vi "SRV_README.vi"   [LabVIEW 2009]
doc: "Contains all the code for the SRV application. <B>This VI is not intended to be run.</B>\n\n\nAuthor: Mike Schultz - Logic PD"
uses:
  SRV VIs/PacketMode/SRV_PM_Packet.ctl
  SRV VIs/TCP_Communication/SRV_TCP Settings.ctl
  SRV VIs/TCP_Communication/SRV_Package Methods.ctl
  SRV VIs/Support/SRV_Command-Data Queue Data Type.ctl
  SRV VIs/ImageProcessing/QT_Image.ctl
  SRV VIs/SubVIs/SRVGlobals.vi
panel:
  # "SRV\nREADME"
types:
  T1 = typedef "SRV_TCP Settings.ctl" = cluster{"Method":T2, "bytes to read":i32, "timeout ms (1000)":i32}
  T2 = typedef "SRV_Package Methods.ctl" = enum16{"General", "Standard", "CRLF", "Image", "HTML"}
  T3 = typedef "Semaphore RefNum" = refnum<k1>
  T4 = typedef "QT_Image.ctl" = cluster{"Witdh":i32, "Height":i32, "Depth":i32, "data":u8[], "Compressed data":u8[], "Color table":u32[], "Duration":i32, "Options":i32, "Timestamp":i32, "ID":i32, "Reserved":i32, "Dialogs":u32}
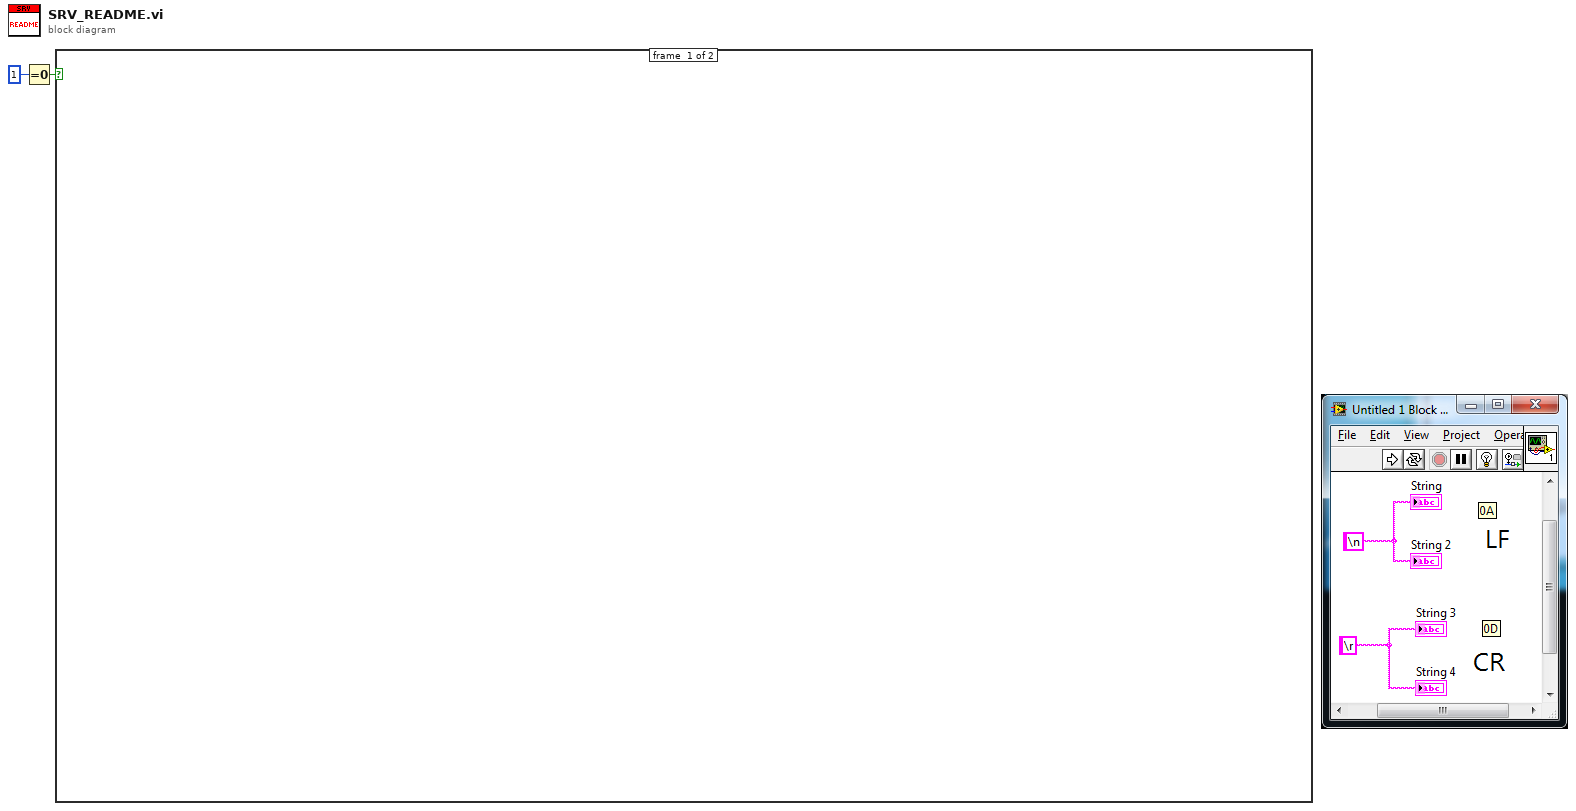
[diagram p0: block diagram]
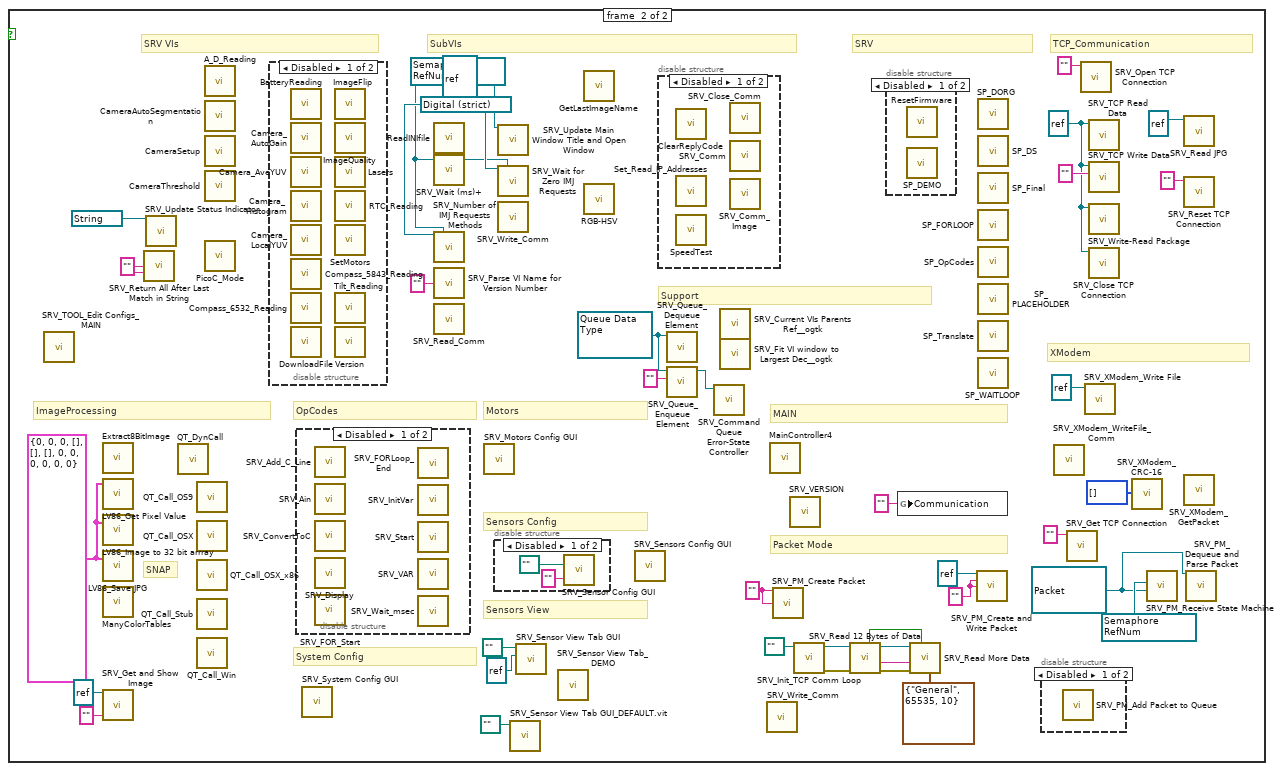
[diagram p2: hidden frame]
diagram:
  n1 = Equal To 0?(x=1) -> (x = 0?=w1:bool)
  n2 = case shown="True" w1 {
    frame #0 {
    }
    frame #1 {
      w6 = refnum<queue> refnum ("SRV_Packets queue")
      w10 = T3 refnum items=["semaphore"] ("TCP Read semaphore")
      w13 = "" ("Command Type")
      w15 = "" ("Command Type")
      w23 = T3 refnum items=["semaphore"] ("semaphore ref")
      w26 = refnum<k5> refnum ("connection ID in")
      w31 = "" ("Reply to XModem Upload")
      w33 = refnum<vi> refnum ("Number of IMJ Requests ref")
      w38 = refnum<queue> refnum ("Command-Data Queue")
      w39 = T4 {"Witdh"=0, "Height"=0, "Depth"=0, "data"=[], "Compressed data"=[], "Color table"=[], "Duration"=0, "Options"=0, "Timestamp"=0, "ID"=0, "Reserved"=0, "Dialogs"=0} ("Image")
      # "SNAP"
      # "MAIN"
      # "System Config"
      # "Sensors View"
      # "Sensors Config"
      # "Motors"
      # "Packet Mode"
      # "TCP_Communication"
      # "XModem"
      # "Support"
      # "SRV"
      # "SubVIs"
      # "SRV VIs"
      # "OpCodes"
      # "ImageProcessing"
      n3 = call "SRV_TOOL_Edit Configs_MAIN.vi"() -> ()  [unwired: 11 in, 1 out]
      n4 = call "Extract8BitImage.vi"() -> ()  [unwired: 2 in, 2 out]
      n5 = call "LV86_Get Pixel Value.vi"("Image In"=w39) -> ()  [unwired: 2 in, 3 out]
      n6 = call "LV86_Image to 32 bit arrray.vi"("Image In"=w39) -> ()  [unwired: 1 in, 2 out]
      n7 = call "LV86_Save JPG.vi"("Image"=w39) -> ()  [unwired: 2 in, 1 out]
      n8 = call "ManyColorTables.vi"() -> ()  [unwired: 3 in, 1 out]
      n9 = call "SRV_Get and Show Image.vi"("Connection ID"=refnum<k5> refnum, "Data"="") -> ()  [unwired: 9 in, 5 out]
      n10 = call "SRV_Return All After Last Match in String.vi"("String"=w31, "String to Match"=w31) -> ()  [unwired: 13 in, 1 out]
      n11 = call "SRV_Update Status Indicator.vi"("Status ref"=refnum<vi> refnum) -> ()  [unwired: 13 in, 2 out]
      n12 = call "QT_DynCall.vi"() -> ()  [unwired: 12 in, 16 out]
      n13 = call "QT_Call_OS9.vi"() -> ()  [unwired: 13 in, 7 out]
      n14 = call "QT_Call_OSX.vi"() -> ()  [unwired: 13 in, 7 out]
      n15 = call "QT_Call_OSX_x86.vi"() -> ()  [unwired: 13 in, 7 out]
      n16 = call "QT_Call_Stub.vi"() -> ()  [unwired: 13 in, 7 out]
      n17 = call "QT_Call_Win.vi"() -> ()  [unwired: 13 in, 7 out]
      n18 = call "A_D_Reading.vi"() -> ()  [unwired: 8 in, 4 out]
      n19 = call "CameraAutoSegmentation.vi"() -> ()  [unwired: 10 in, 2 out]
      n20 = call "CameraSetup.vi"() -> ()  [unwired: 10 in, 2 out]
      n21 = call "CameraThreshold.vi"() -> ()  [unwired: 10 in, 2 out]
      n22 = call "PicoC_Mode.vi"() -> ()  [unwired: 10 in, 2 out]
      n23 = disable-structure shown="Disabled" {
        frame #0 {
          n24 = call "BatteryReading.vi"() -> ()  [unwired: 3 in, 2 out]
          n25 = call "Camera_AutoGain.vi"() -> ()  [unwired: 3 in, 2 out]
          n26 = call "Camera_AveYUV.vi"() -> ()  [unwired: 3 in, 2 out]
          n27 = call "Camera_Histogram.vi"() -> ()  [unwired: 4 in, 1 out]
          n28 = call "Camera_LocalYUV.vi"() -> ()  [unwired: 3 in, 2 out]
          n29 = call "Compass_5843_Reading.vi"() -> ()  [unwired: 3 in, 2 out]
          n30 = call "Compass_6532_Reading.vi"() -> ()  [unwired: 3 in, 2 out]
          n31 = call "DownloadFile.vi"() -> ()  [unwired: 10 in, 2 out]
          n32 = call "ImageFlip.vi"() -> ()  [unwired: 4 in, 1 out]
          n33 = call "ImageQuality.vi"() -> ()  [unwired: 4 in, 1 out]
          n34 = call "Lasers.vi"() -> ()  [unwired: 4 in, 1 out]
          n35 = call "RTC_Reading.vi"() -> ()  [unwired: 3 in, 2 out]
          n36 = call "SetMotors.vi"() -> ()  [unwired: 5 in, 2 out]
          n37 = call "Tilt_Reading.vi"() -> ()  [unwired: 3 in, 2 out]
          n38 = call "Version.vi"() -> ()  [unwired: 8 in, 4 out]
        }
        frame #1 {
        }
      }
      n39 = disable-structure shown="Disabled" {
        frame #0 {
          n40 = call "SRV_Add_C_Line.vi"() -> ()  [unwired: 5 in, 1 out]
          n41 = call "SRV_Ain.vi"() -> ()  [unwired: 3 in, 2 out]
          n42 = call "SRV_ConvertToC.vi"() -> ()  [unwired: 2 in, 2 out]
          n43 = call "SRV_Display.vi"() -> ()  [unwired: 4 in, 1 out]
          n44 = call "SRV_FOR_Start.vi"() -> ()  [unwired: 3 in, 2 out]
          n45 = call "SRV_FORLoop_End.vi"() -> ()  [unwired: 4 in, 1 out]
          n46 = call "SRV_InitVar.vi"() -> ()  [unwired: 2 in, 1 out]
          n47 = call "SRV_Start.vi"() -> ()  [unwired: 4 in, 1 out]
          n48 = call "SRV_VAR.vi"() -> ()  [unwired: 3 in, 4 out]
          n49 = call "SRV_Wait_msec.vi"() -> ()  [unwired: 4 in, 1 out]
        }
        frame #1 {
        }
      }
      n50 = call "SRV_System Config GUI.vi"() -> ()  [unwired: 9 in, 3 out]
      n51 = call "ReadINIfile.vi"() -> ()  [unwired: 9 in, 3 out]
      n52 = call "SRV_Wait (ms)+.vi"() -> ()  [unwired: 14 in, 2 out]
      n53 = call "SRV_Number of IMJ Requests Methods.vi"("Number of IMJ Requests ref"=w33, "semaphore ref"=w23) -> ()  [unwired: 9 in, 5 out]
      n54 = call "SRV_Parse VI Name for Version Number.vi"("VI Name"="") -> ()  [unwired: 14 in, 1 out]
      n55 = call "SRV_Read_Comm.vi"() -> ()  [unwired: 9 in, 3 out]
      n56 = call "SRV_Motors Config GUI.vi"() -> ()  [unwired: 9 in, 3 out]
      n57 = disable-structure shown="Disabled" {
        frame #0 {
          n58 = call "SRV_Sensor Config GUI.vi"("Sensor to Edit"="", "Sensors Config File Path in"=path "") -> ()  [unwired: 7 in, 3 out]
        }
        frame #1 {
        }
      }
      n59 = call "SRV_Update Main Window Title and Open Window.vi"("VI ref"=refnum<vi> refnum) -> ()  [unwired: 13 in, 2 out]
      n60 = call "SRV_Wait for Zero IMJ Requests.vi"("Number of IMJ Requests ref"=w33, "#IMJ semaphore ref"=w23) -> ()  [unwired: 11 in, 3 out]
      n61 = call "SRV_Write_Comm.vi"() -> ()  [unwired: 9 in, 3 out]
      n62 = call "SRV_Sensor View Tab GUI_DEFAULT.vit"("Sensors Config File Path"=path "") -> ()  [unwired: 10 in, 1 out]
      n63 = call "SRV_Sensor View Tab GUI.vi"("SRV In"=refnum<k5> refnum, "Sensors Config File Path"=path "") -> ()  [unwired: 9 in, 1 out]
      n64 = call "SRV_Sensor View Tab_DEMO.vi"() -> ()  [unwired: 1 in]
      n65 = call "GetLastImageName.vi"() -> ()  [unwired: 1 in, 1 out]
      n66 = call "RGB-HSV.vi"() -> ()  [unwired: 14 in, 2 out]
      n67 = call "SRV_Sensors Config GUI.vi"() -> ()  [unwired: 9 in, 3 out]
      n68 = disable-structure shown="Disabled" {
        frame #0 {
          n69 = call "ClearReplyCode.vi"() -> ()  [unwired: 1 in, 1 out]
          n70 = call "Set_Read_IP_Addresses.vi"() -> ()  [unwired: 3 in, 1 out]
          n71 = call "SpeedTest.vi"() -> ()  [unwired: 1 in]
          n72 = call "SRV_Close_Comm.vi"() -> ()  [unwired: 9 in, 3 out]
          n73 = call "SRV_Comm.vi"() -> ()  [unwired: 3 in, 3 out]
          n74 = call "SRV_Comm_Image.vi"() -> ()  [unwired: 3 in, 3 out]
        }
        frame #1 {
        }
      }
      n75 = call "SRV_Queue_Dequeue Element.vi"("Command-Data Queue"=w38) -> ()  [unwired: 5 in, 6 out]
      n76 = call "SRV_Queue_Enqueue Element.vi"("Command"="", "Command-Data Queue"=w38) -> ("Command-Data Queue out"=w22:refnum<queue>)  [unwired: 7 in, 2 out]
      n77 = call "SRV_Command Queue Error-State Controller.vi"("Command-Data Queue"=w22) -> ()  [unwired: 9 in, 2 out]
      n78 = call "SRV_Current VIs Parents Ref__ogtk.vi"() -> ()  [unwired: 2 in, 1 out]
      n79 = call "SRV_Fit VI window to Largest Dec__ogtk.vi"() -> ()  [unwired: 6 in, 2 out]
      n80 = call "SRV_Write_Comm.vi"() -> ()  [unwired: 9 in, 3 out]
      n81 = call "MainController4.vi"() -> ()  [unwired: 1 in]
      n82 = call "SRV_PM_Create Packet.vi"("Command Type"=w15, "Data String"=w15) -> ()  [unwired: 12 in, 2 out]
      n83 = call "SRV_VERSION.vi"() -> ()  [unwired: 1 out]
      n84 = call "SRV_Init_TCP Comm Loop.vi"("System Config File Path in"=path "") -> ("error out"=w16:errorcluster, "connection ID"=w17:refnum<k5>)  [unwired: 7 in, 2 out]
      n85 = call "SRV_Read 12 Bytes of Data.vi"("error in (no error)"=w16, "SRV In"=w17) -> ("error out"=w20:errorcluster, "Data out"=w21:string, "SRV Out"=w19:refnum<k5>, "Read more data"=w18:bool)  [unwired: 6 in]
      n86 = disable-structure shown="Disabled" {
        frame #0 {
          n87 = call "ResetFirmware.vi"() -> ()  [unwired: 3 in, 3 out]
          n88 = call "SP_DEMO.vi"() -> ()  [unwired: 1 in]
        }
        frame #1 {
        }
      }
      n89 = global write "SRVGlobals.vi" "Communication"("" ("Communication")) -> ()
      n90 = call "SRV_Read More Data.vi"("TCP Settings"=T1 {"Method"=enum."General", "bytes to read"=65535, "timeout ms (1000)"=10}, "Read More Data? (T)"=w18, "error in (no error)"=w20, "Data in"=w21, "Connection ID"=w19) -> ()  [unwired: 4 in, 3 out]
      n91 = call "SRV_PM_Create and Write Packet.vi"("SRV ref"=refnum<k5> refnum, "Command Type"=w13, "Data String"=w13) -> ()  [unwired: 11 in, 2 out]
      n92 = call "SP_DORG.vi"() -> ()  [unwired: 3 in, 1 out]
      n93 = call "SP_DS.vi"() -> ()  [unwired: 3 in, 1 out]
      n94 = call "SP_Final.vi"() -> ()  [unwired: 2 in, 1 out]
      n95 = call "SP_FORLOOP.vi"() -> ()  [unwired: 3 in, 1 out]
      n96 = call "SP_OpCodes.vi"() -> ()  [unwired: 3 in, 1 out]
      n97 = call "SP_PLACEHOLDER.vi"() -> ()  [unwired: 3 in, 1 out]
      n98 = call "SP_Translate.vi"() -> ()  [unwired: 3 in, 1 out]
      n99 = call "SP_WAITLOOP.vi"() -> ()  [unwired: 3 in, 1 out]
      n100 = disable-structure shown="Disabled" {
        frame #0 {
          n101 = call "SRV_PM_Add Packet to Queue.vi"() -> ()  [unwired: 15 in, 1 out]
        }
        frame #1 {
        }
      }
      n102 = call "SRV_XModem_WriteFile_Comm.vi"() -> ()  [unwired: 7 in, 5 out]
      n103 = call "SRV_Get TCP Connection.vi"("IP address"="") -> ()  [unwired: 9 in, 2 out]
      n104 = call "SRV_Open TCP Connection.vi"("IP address"="") -> ()  [unwired: 9 in, 2 out]
      n105 = call "SRV_XModem_Write File.vi"("connection ID in"=refnum<k5> refnum) -> ()  [unwired: 6 in, 5 out]
      n106 = call "SRV_TCP Read Data.vi"("connection ID in"=w26) -> ()  [unwired: 4 in, 4 out]
      n107 = call "SRV_TCP Write Data.vi"("data in"="", "connection ID"=w26) -> ()  [unwired: 7 in, 3 out]
      n108 = call "SRV_Write-Read Package.vi"("connection ID in"=w26) -> ()  [unwired: 7 in, 4 out]
      n109 = call "SRV_Close TCP Connection.vi"("connection ID"=w26) -> ()  [unwired: 10 in, 1 out]
      n110 = call "SRV_XModem_CRC-16.vi"("Array"=u8[] []) -> ()  [unwired: 14 in, 1 out]
      n111 = call "SRV_PM_Receive State Machine.vi"("SRV_Packets queue"=w6, "TCP Read semaphore"=w10) -> ()  [unwired: 9 in, 1 out]
      n112 = call "SRV_Read JPG.vi"("connection ID in"=refnum<k5> refnum) -> ()  [unwired: 8 in, 3 out]
      n113 = call "SRV_Reset TCP Connection.vi"("IP address"="") -> ()  [unwired: 9 in, 2 out]
      n114 = call "SRV_XModem_GetPacket.vi"() -> ()  [unwired: 4 in, 1 out]
      n115 = call "SRV_PM_Dequeue and Parse Packet.vi"("SRV_Packets queue"=w6) -> ()  [unwired: 5 in, 10 out]
    }
  }
